vi "Determine State.vi"(8 "error in":errorcluster, 11 "Fault Handler in":refnum<class "Fault Handler.lvclass">) -> (0 "error out":errorcluster, 1 "Nominal":bool, 3 "Fault Handler out":refnum<class "Fault Handler.lvclass">, 4 "Error State":T1)   [LabVIEW 2019, in "Fault Handler.lvlib" / "Fault Handler.lvclass"]
doc: "This routine inspects active alarm and active warning records and prioritizes a status update based on the state of the system:\n\n<b>No Fault Present</b>\nNominal Flag == <b>TRUE</b>\nError State == <b>Previous</b>\n\n<b>Error Present</b>\nNominal Flag == <b>FALSE</b>\nError State == <b>Error</b>\n\n<b>Warning Present</b>\nNominal Flag == <b>FALSE</b>\nError State == <b>Warning</b>\n\n<b>Error & Warning Fault Present</b>\nNominal Flag == <b>FALSE</b>\nError State == <b>Error</b>"
uses:
  Project/Fault Handler.lvclass
  builds/Engine/Engine.lvlibp/Custom Controls/System Status.ctl
  Project/Fault Handler.lvclass/Fault Handler.ctl
  builds/Engine/Engine.lvlibp/Project/Engine.lvclass
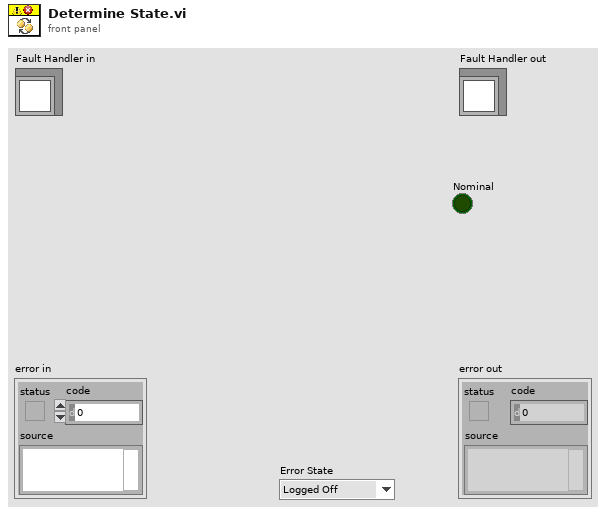
[diagram p1: front panel]
types:
  T1 = typedef "Engine.lvlibp/Engine.lvclass/System Status.ctl" = enum16{"Logged Off", "UUT_Info_Missing", "Idle", "Error", "Warning", "Loading", "Config", "Manual", "Automation", "Report_View", "Previous"}
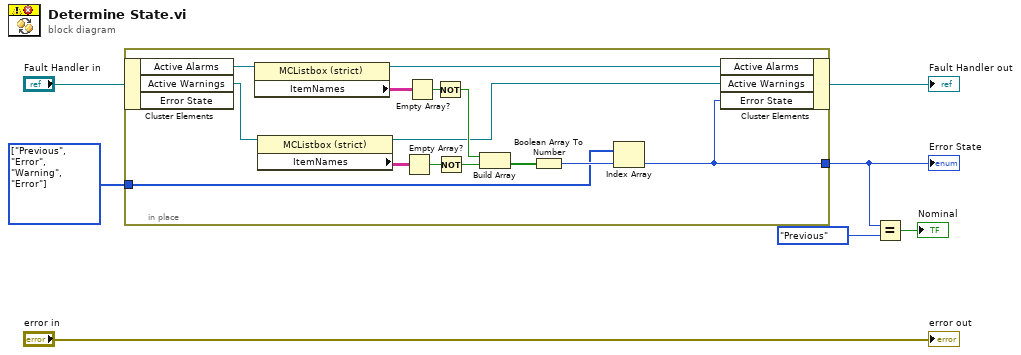
[diagram p0: block diagram]
diagram:
  w4 = T1[] [enum."Previous", enum."Error", enum."Warning", enum."Error"] items=["Logged Off", "UUT_Info_Missing", "Idle", "Error", "Warning", "Loading", "Config", "Manual", "Automation", "Report_View", "Previous"]
  n1 = in-place {
    in-place-border: w4 -> [w9]
    in-place-border: [w8] -> w3
    n2 = in-place-cluster #1("Fault Handler in") -> ("Active Alarms"=w15:refnum<vi>, "Active Warnings"=w13:refnum<vi>)  [unwired: 1 out]
    n3 = property class="MCListbox (strict)"(reference=w15) -> (reference out=w14:refnum<vi>, "ItemNames"=w17:string[][])  [unwired: 1 in, 1 out]
    n4 = property class="MCListbox (strict)"(reference=w13) -> (reference out=w12:refnum<vi>, "ItemNames"=w16:string[][])  [unwired: 1 in, 1 out]
    n5 = Empty Array?(array=w16) -> (empty?=w19:bool)
    n6 = Empty Array?(array=w17) -> (empty?=w18:bool)
    n7 = Not(x=w18) -> (.not. x?=w20:bool)
    n8 = Not(x=w19) -> (.not. x?=w21:bool)
    n9 = Build Array(w20, w21) -> (w11:bool[])
    n10 = Boolean Array To Number(Boolean array=w11) -> (number=w10:u32)
    n11 = Index Array(array=w9, index=w10) -> (element=w8:T1)
    n12 = in-place-cluster #1("Active Alarms"=w14, "Active Warnings"=w12, "Error State"=w8) -> (→"Fault Handler out":refnum<class "Fault Handler.lvclass">)
  }
  "Error State" <- w3
  n13 = Equal?(x=w3, y=System_Status."Previous") -> (x = y?=→"Nominal":bool)
  "error out" <- "error in"
